vi "Write relativeHumidity_percent.vi"(8 "error in (no error)":errorcluster, 10 "relativeHumidity_percent":dbl=20.0 min=0.0 max=100.0, 11 "WSSet in":refnum<class "WSSet.lvclass">) -> (0 "error out":errorcluster, 3 "WSSet out":refnum<class "WSSet.lvclass">)   [LabVIEW 2022 SP3, in "TCSDataDefinitions.lvlib" / "TCSWeatherServerCommand.lvlib" / "WSSet.lvclass"]
uses:
  WSSet.lvclass
  WSSet.lvclass/WSSet.ctl
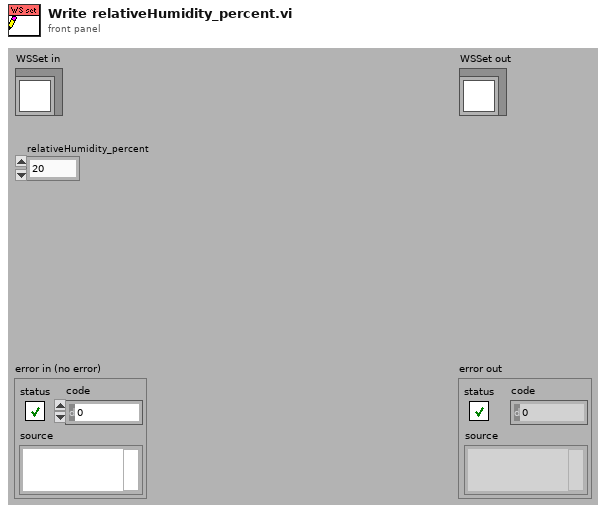
[diagram p1: front panel]
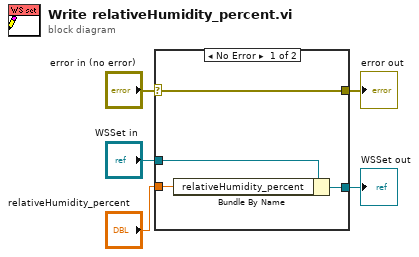
[diagram p0: block diagram]
diagram:
  n1 = case shown="No Error" "error in (no error)" {
    selector: "error in (no error)" -> [w9 w10]
    tunnel: [w9 w10] -> w4
    tunnel: [w7 w11] -> w2
    tunnel: "WSSet in" -> [w8 w11]
    tunnel: "relativeHumidity_percent" -> [w6 _]
    frame No Error {
      n2 = Bundle By Name(cluster=w8, "relativeHumidity_percent"=w6) -> (w7:refnum<class "WSSet.lvclass">)
    }
    frame Error {
    }
  }
  "error out" <- w4
  "WSSet out" <- w2
